vi "npk project.vi"() -> ()   [LabVIEW 2015]
panel:
  in  "stop":bool
  in  "K":dbl
  in  "P":dbl
  in  "N":dbl
  out "OPEN":bool
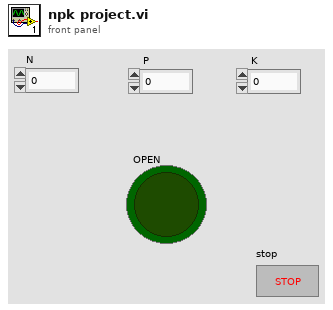
[diagram p1: front panel]
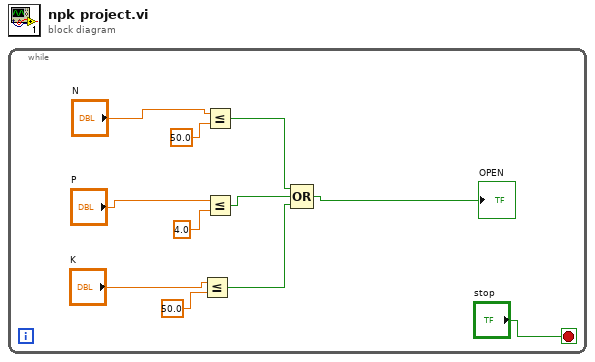
[diagram p0: block diagram]
diagram:
  n1 = while {
    stop <- "stop" stop-if-true
    n2 = Less Or Equal?(x="K", y=50.0 ("x")) -> (x <= y?=w3:bool)
    n3 = Less Or Equal?(x="N", y=50.0) -> (x <= y?=w5:bool)
    n4 = Less Or Equal?(x="P", y=4.0) -> (x <= y?=w4:bool)
    n5 = Compound Arithmetic op=OR(w5, w4, w3) -> (→"OPEN":bool)
  }
